vi "Calculate Overall Status.vi"(8 "error in (no error)":errorcluster, 11 "abs_Parallel in":refnum<class "abs_Parallel.lvclass">) -> (0 "error out":errorcluster, 2 "Overall Status":T1, 3 "abs_Parallel out":refnum<class "abs_Parallel.lvclass">)   [LabVIEW 2021, in "BT.lvlib" / "abs_Parallel.lvclass"]
uses:
  abs_Parallel.lvclass
  abs_Node/Status.ctl
  abs_Parallel.lvclass/abs_Parallel.ctl
  abs_Node/abs_Node.lvclass
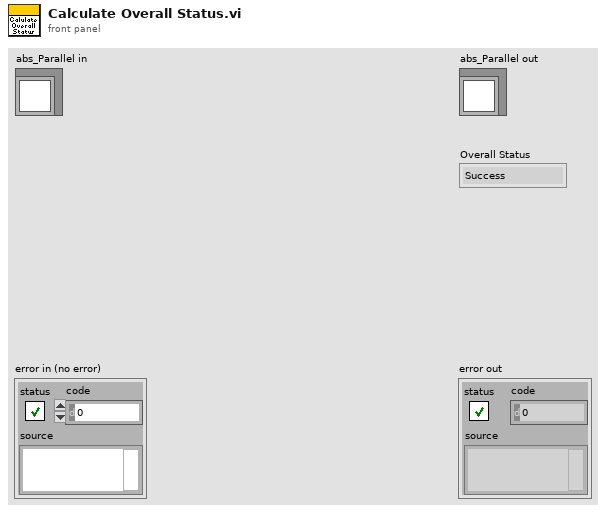
[diagram p1: front panel]
types:
  T1 = typedef "BT.lvlib/abs_Node.lvclass/Status.ctl" = enum16{"Success", "Failure", "Running"}
  T2 = typedef "BT.lvlib/abs_Parallel.lvclass/Status Calculation.ctl" = enum16{"Succeed on All Succeed", "Failure on All Failure", "Succeed on Any Succeed", "Failure on Any Failure"}
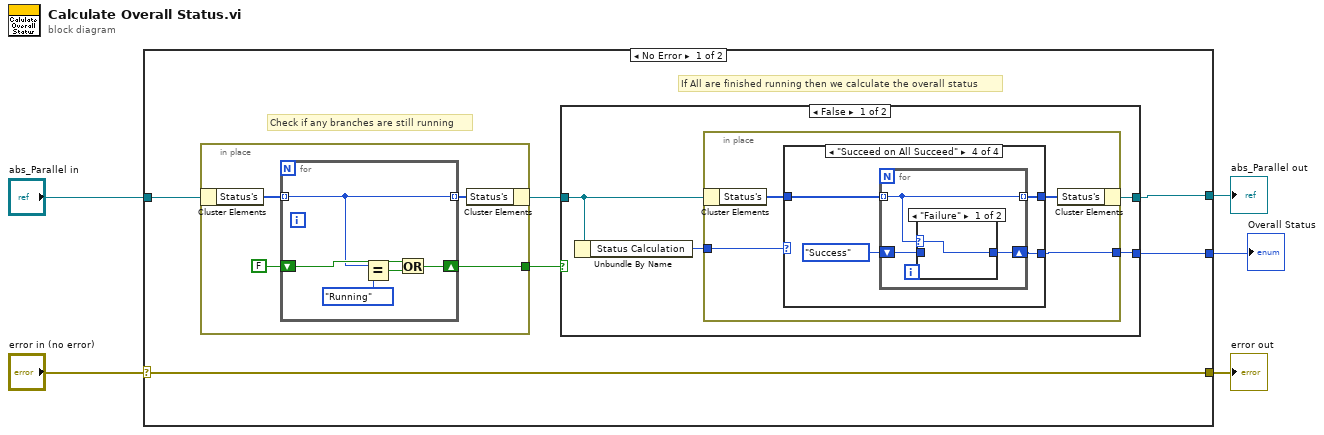
[diagram p0: block diagram]
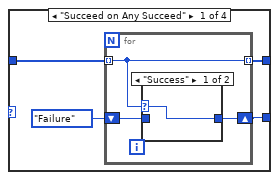
[diagram p2: hidden frame]
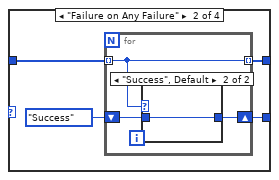
[diagram p4: hidden frame]
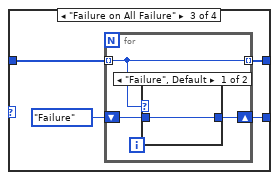
[diagram p6: hidden frame]
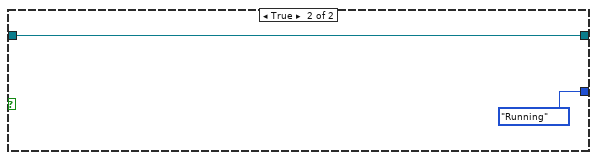
[diagram p9: hidden frame]
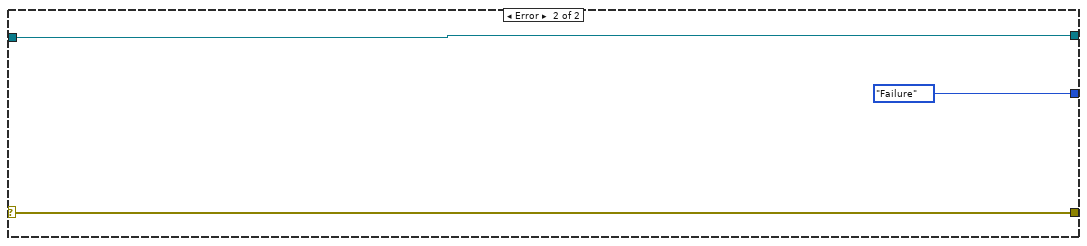
[diagram p10: hidden frame]
diagram:
  n1 = case shown="No Error" "error in (no error)" {
    selector: "error in (no error)" -> [w7 w69]
    tunnel: [w7 w69] -> w4
    tunnel: [w9 w68] -> w2
    tunnel: "abs_Parallel in" -> [w6 w68]
    tunnel: [w8 Status."Failure" ("y")] -> w1
    frame No Error {
      # "If All are finished running then we calculate the overall status"
      # "Check if any branches are still running"
      n2 = in-place {
        in-place-border: [w15] -> w11
        n3 = in-place-cluster #1(w6) -> ("Status's"=w13:T1[])
        n4 = for {
          tunnel: w13 -> [w16] mode=indexing
          shift-right: [w19] -> w15
          shift-left: FALSE -> [w18]
          tunnel: [w16] -> w12 mode=indexing
          n5 = Equal?(x=w16, y=Status."Running") -> (x = y?=w17:bool)
          n6 = Or(x=w18, y=w17) -> (x .or. y?=w19:bool)
        }
        n7 = in-place-cluster #1("Status's"=w12) -> (w10:refnum<class "abs_Parallel.lvclass">)
      }
      n8 = case shown="False" w11 {
        tunnel: [w21 Status."Running" ("y")] -> w8
        tunnel: w10 -> [w23 w65]
        tunnel: [w24 w65] -> w9
        frame False {
          n9 = Unbundle By Name(w23) -> ("Status Calculation"=w22:T2)
          n10 = in-place {
            in-place-border: w22 -> [w26]
            in-place-border: [w25] -> w21
            n11 = in-place-cluster #2(w23) -> ("Status's"=w28:T1[])
            n12 = case shown="\"Succeed on All Succeed\"" w26 {
              tunnel: w28 -> [w32 w41 w50 w59]
              tunnel: [w31 w40 w49 w58] -> w27
              tunnel: [w30 w39 w48 w57] -> w25
              frame "Succeed on Any Succeed" {
                n13 = for {
                  tunnel: w32 -> [w35] mode=indexing
                  tunnel: [w35] -> w31 mode=indexing
                  shift-right: [w34] -> w30
                  shift-left: Status."Failure" ("Status") -> [w33]
                  n14 = case shown="\"Success\"" w35 {
                    selector: w35 -> [w36 _]
                    tunnel: [w36 w37] -> w34
                    tunnel: w33 -> [_ w37]
                    frame "Success" {
                    }
                    frame "Failure", Default {
                    }
                  }
                }
              }
              frame "Failure on Any Failure" {
                n15 = for {
                  tunnel: w41 -> [w44] mode=indexing
                  tunnel: [w44] -> w40 mode=indexing
                  shift-right: [w43] -> w39
                  shift-left: Status."Success" ("Status") -> [w42]
                  n16 = case shown="\"Success\", Default" w44 {
                    selector: w44 -> [w45 _]
                    tunnel: [w45 w46] -> w43
                    tunnel: w42 -> [_ w46]
                    frame "Failure" {
                    }
                    frame "Success", Default {
                    }
                  }
                }
              }
              frame "Failure on All Failure" {
                n17 = for {
                  tunnel: w50 -> [w53] mode=indexing
                  tunnel: [w53] -> w49 mode=indexing
                  shift-right: [w52] -> w48
                  shift-left: Status."Failure" ("Status") -> [w51]
                  n18 = case shown="\"Failure\", Default" w53 {
                    selector: w53 -> [_ w55]
                    tunnel: [w54 w55] -> w52
                    tunnel: w51 -> [w54 _]
                    frame "Failure", Default {
                    }
                    frame "Success" {
                    }
                  }
                }
              }
              frame "Succeed on All Succeed" {
                n19 = for {
                  tunnel: w59 -> [w62] mode=indexing
                  tunnel: [w62] -> w58 mode=indexing
                  shift-right: [w61] -> w57
                  shift-left: Status."Success" ("Status") -> [w60]
                  n20 = case shown="\"Failure\"" w62 {
                    selector: w62 -> [w63 _]
                    tunnel: [w63 w64] -> w61
                    tunnel: w60 -> [_ w64]
                    frame "Failure" {
                    }
                    frame "Success", Default {
                    }
                  }
                }
              }
            }
            n21 = in-place-cluster #2("Status's"=w27) -> (w24:refnum<class "abs_Parallel.lvclass">)
          }
        }
        frame True {
        }
      }
    }
    frame Error {
    }
  }
  "error out" <- w4
  "abs_Parallel out" <- w2
  "Overall Status" <- w1
